vi "Insert Private VIs.vi"(4 "New Node Name":string="Errors", 6 "pattern":string, 7 "Application in":refnum<vi>, 8 "Tree Map in":T1, 9 "Root path":string, 10 "DQMH Lib In":refnum<vi>) -> (0 "Tree Map Out":T1)   [LabVIEW 2019, in "Panther Dashboard.lvlib"]
uses:
  Panther Dashboard.lvlib
  <vilib>/National Instruments/Tree Map/Tree Map Data.ctl
  Map Attribute--enum.ctl
  <vilib>/National Instruments/Tree Map/Tree Map.lvlib
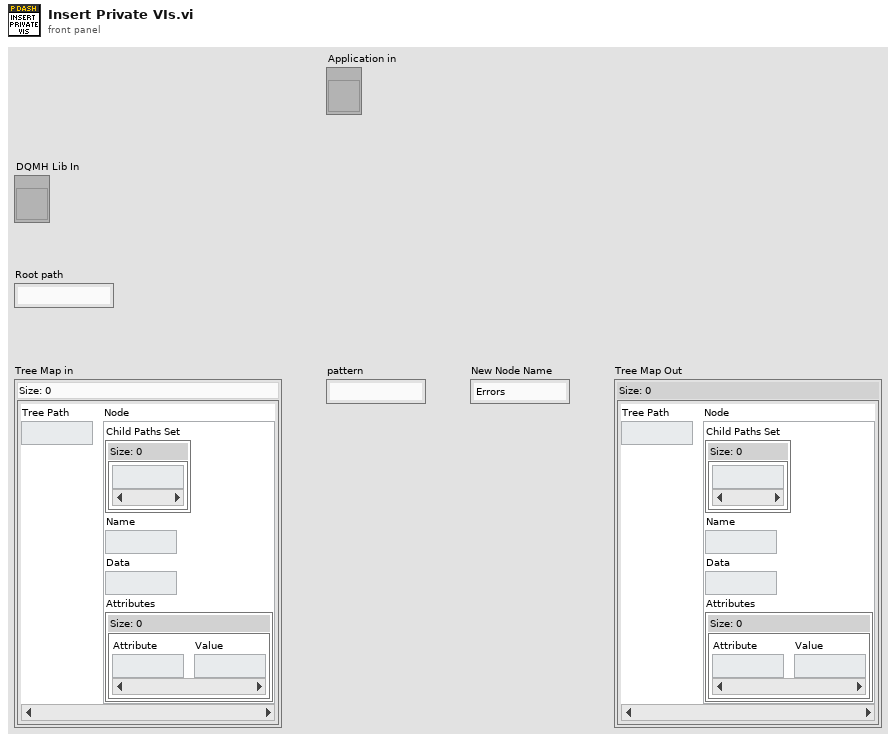
[diagram p1: front panel]
types:
  T1 = typedef "Tree Map.lvlib/Tree Map Data.ctl" = map{string, cluster{"Child Paths Set":set{string}, "Name":string, "Data":string, "Attributes":map{string, string}}}
  T2 = typedef "Panther Dashboard.lvlib/Map Attribute--enum.ctl" = enum16{"Path", "ModuleType", "Module Description", "Dependency?", "Target"}
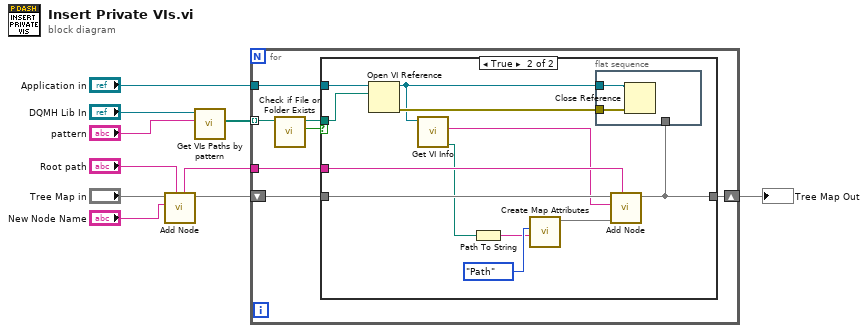
[diagram p0: block diagram]
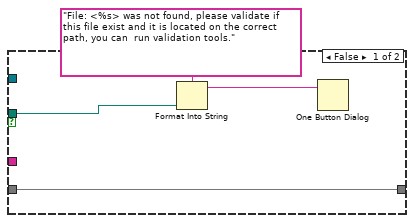
[diagram p2: hidden frame]
diagram:
  n1 = call <vilib>:"Add Node.vi"("Parent Path"="Root path", "New Node Name"="New Node Name", "Tree Map In"="Tree Map in") -> ("Tree Map Out"=w6:T1, "New Node Path"=w4:string)  [unwired: 6 in, 1 out]
  n2 = call "Get VIs Paths by pattern.vi"("pattern"="pattern", "Library in"="DQMH Lib In") -> ("All Files in Dir"=w2:path[])  [unwired: 7 in, 2 out]
  n3 = for {
    tunnel: "Application in" -> [w17]
    shift-right: [w16] -> w9
    shift-left: w6 -> [w15]
    tunnel: w4 -> [w14]
    tunnel: w2 -> [w11] mode=indexing
    n4 = call <vilib>:"Check if File or Folder Exists.vi"("path"=w11) -> ("file or folder exists?"=w13:bool, "dup path"=w12:path)  [unwired: 8 in, 1 out]
    n5 = case shown="True" w13 {
      tunnel: w17 -> [_ w32]
      tunnel: [w21 w22] -> w16
      tunnel: w15 -> [w21 w31]
      tunnel: w14 -> [_ w30]
      tunnel: w12 -> [w20 w28]
      frame False {
        n6 = Format Into String(format string="File: <%s> was not found, please validate if this file exist and it is located on the correct path, you can  run validation tools.", w20) -> (resulting string=w19:string)  [unwired: 2 in, 1 out]
        n7 = One Button Dialog(message=w19) -> ()  [unwired: 1 in, 1 out]
      }
      frame True {
        n8 = Open VI Reference(application reference (local)=w32, vi path=w28) -> (vi reference=w23:refnum<vi>, error out=w33:errorcluster)  [unwired: 4 in]
        n9 = call "Get VI Info.vi"("VI in"=w23) -> ("VI Path"=w24:path, "Plain Name"=w29:string)  [unwired: 7 in, 2 out]
        n10 = Path To String(path=w24) -> (string=w26:string)
        n11 = call "Create Map Attributes.vi"("Attribute"=w26, "Map Attribute"=Map_Attribute--enum."Path") -> ("Root Attributes"=w25:map{string, string})  [unwired: 9 in]
        n12 = flat-sequence {
          tunnel: w33 -> [w35]
          tunnel: w23 -> [w34]
          tunnel: w22 -> [_]
          frame #0 {
            n13 = Close Reference(reference=w34, error in (no error)=w35) -> ()  [unwired: 1 out]
          }
        }
        n14 = call <vilib>:"Add Node.vi"("Parent Path"=w30, "Attributes"=w25, "New Node Name"=w29, "Tree Map In"=w31) -> ("Tree Map Out"=w22:T1)  [unwired: 5 in, 2 out]
      }
    }
  }
  "Tree Map Out" <- w9
